vi "Count Edges.vi"(11 "Positions":map{T3, bool[]}(c390)) -> (3 "size(s)":i32)   [LabVIEW 2024]
uses:
  Utility/Universal Utility/TypeDefs_Utility/Cluster_Row-Column.ctl
  Cluster_Side Datactl.ctl
  Utility/Universal Utility/TypeDefs_Utility/ENUM_4 Directions U-D-L-R.ctl
panel:
  out "Edges":T1[](array[typedef])
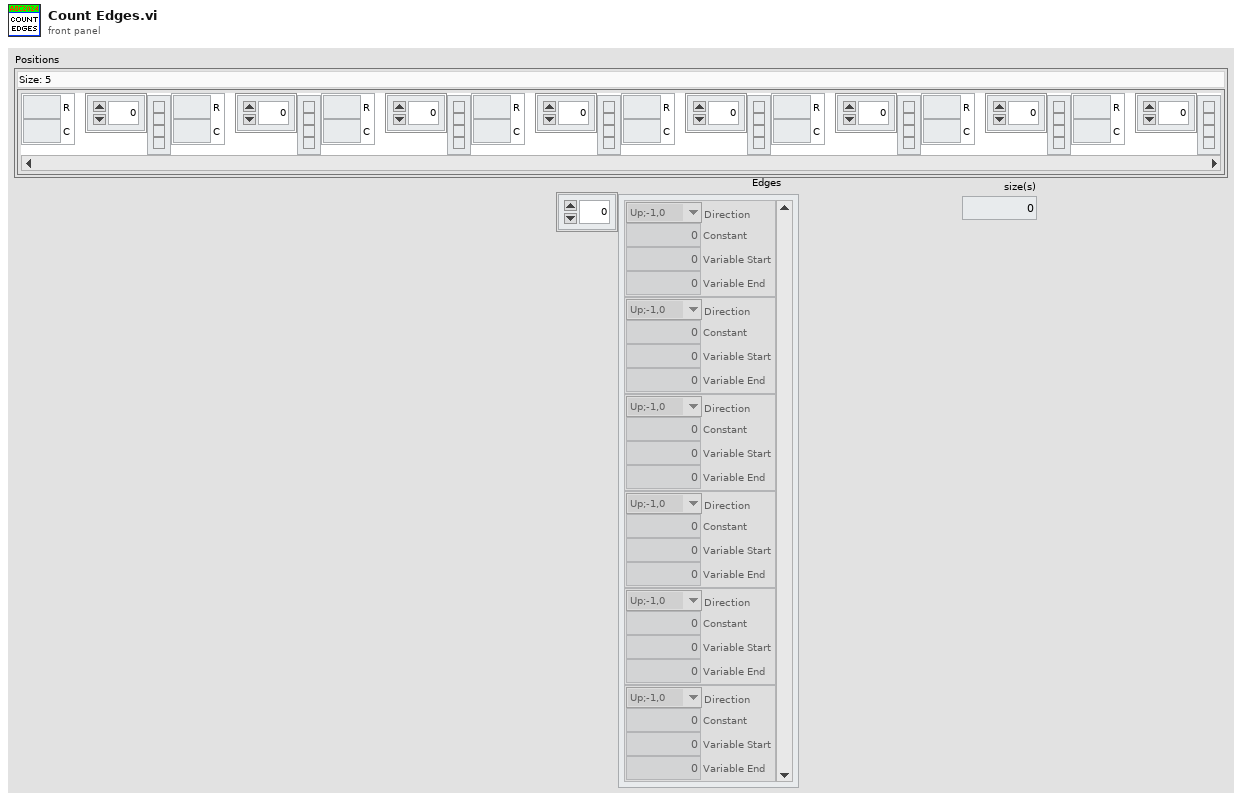
[diagram p1: front panel]
types:
  T1 = typedef "Cluster_Side Datactl.ctl" = cluster{"Direction":T2, "Constant":i32, "Variable Start":i32, "Variable End":i32}
  T2 = typedef "ENUM_4 Directions U-D-L-R.ctl" = enum16{"Up;-1,0", "Right;0,1", "Down;1,0", "Left;0,-1"}
  T3 = typedef "Cluster_Row-Column.ctl" = cluster{"R":i32, "C":i32}
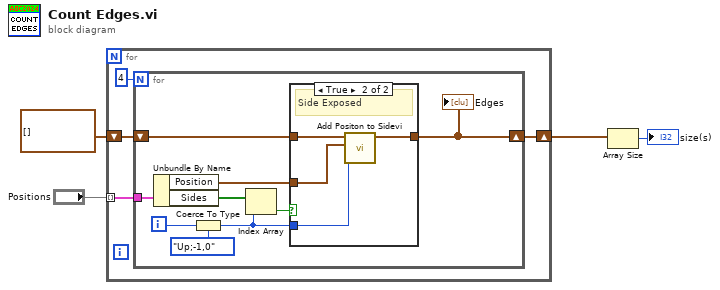
[diagram p0: block diagram]
diagram:
  n1 = for {
    tunnel: "Positions" -> [w8] mode=indexing
    shift-right: [w6] -> w2
    shift-left: T1[] [] ("Left Right") -> [w7]
    n2 = for {
      N: 4 -> [_]
      tunnel: w8 -> [w17]
      shift-right: [w9] -> w6
      shift-left: w7 -> [w13]
      i -> [w10]
      n3 = Unbundle By Name(w17) -> ("Position"=w14:T3, "Sides"=w16:bool[])
      n4 = Coerce To Type(0:w10, 1:ENUM_4_Directions_U-D-L-R."Up;-1,0" ("Direction")) -> (2:w11:T2)
      n5 = Index Array(array=w16, index=w11) -> (element=w15:bool)
      n6 = case shown="True" w15 {
        tunnel: w14 -> [_ w20]
        tunnel: w11 -> [_ w22]
        tunnel: w13 -> [w18 w21]
        tunnel: [w18 w19] -> w9
        frame False {
          # "Side Not Exposed"
        }
        frame True {
          # "Side Exposed"
          n7 = call "Add Positon to Sidevi.vi"("Direction"=w22, "Position"=w20, "Side Array"=w21) -> ("Side Array Out"=w19:T1[])  [unwired: 8 in]
        }
      }
      "Edges" <- w9
    }
  }
  n8 = Array Size(array=w2) -> (size(s)=→"size(s)":i32)
